vi "Encrypts.vi"(8 "error in (no error)":errorcluster caption="entrée d'erreur (pas d'erreur)", 11 "Cryptographic Hash_SHA256 en entrée":refnum<class "Cryptographic Hash_SHA256.lvclass">) -> (0 "error out":errorcluster caption="sortie d'erreur", 3 "Cryptographic Hash_SHA256 en sortie":refnum<class "Cryptographic Hash_SHA256.lvclass">)   [LabVIEW 2020, in "Library Cryptographic Hash.lvlib" / "Cryptographic Hash_SHA256.lvclass"]
uses:
  Cryptographic Hash_SHA256.lvclass
  C:/Users/ngarcin/OneDrive - Altyor/Standard TB/Class/Cryptographic Hash/Cryptographic Hash (Default)/Cryptographic Hash (Default).lvclass
  Cryptographic Hash_SHA256.lvclass/Cryptographic Hash_SHA256.ctl
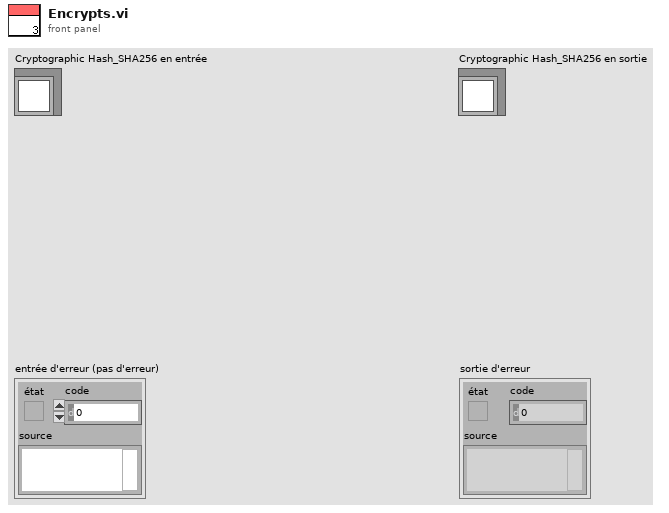
[diagram p1: front panel]
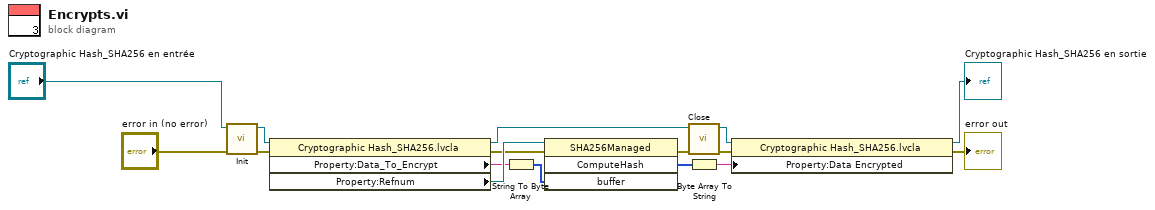
[diagram p0: block diagram]
diagram:
  n1 = call-dynamic "Init.vi"("error in (no error)"="error in (no error)", "Cryptographic Hash_SHA256 en entrée"="Cryptographic Hash_SHA256 en entrée") -> ("error out"=w12:errorcluster, "Cryptographic Hash_SHA256 en sortie"=w13:refnum<class "Cryptographic Hash_SHA256.lvclass">)  [unwired: 8 in]
  n2 = property class="Cryptographic Hash_SHA256.lvcla"(reference=w13, error in=w12) -> (reference out=w10:refnum<class "Cryptographic Hash_SHA256.lvclass">, error out=w2:errorcluster, "Property:Data_To_Encrypt"=w3:string, "Property:Refnum"=w4:refnum<k24>)
  n3 = String To Byte Array(string=w3) -> (unsigned byte array=w16:u8[])
  n4 = invoke class="SHA256Managed" method="ComputeHash"(reference=w4, error in=w2, "buffer"=w16) -> (error out=w1:errorcluster, "ComputeHash"=w15:u8[])  [unwired: 1 in, 2 out]
  n5 = call-dynamic "Close.vi"("error in (no error)"=w1, "Cryptographic Hash_SHA256 en entrée"=w10) -> ("error out"=w6:errorcluster, "Cryptographic Hash_SHA256 en sortie"=w9:refnum<class "Cryptographic Hash_SHA256.lvclass">)  [unwired: 8 in]
  n6 = Byte Array To String(unsigned byte array=w15) -> (string=w7:string)
  n7 = property class="Cryptographic Hash_SHA256.lvcla"(reference=w9, error in=w6, "Property:Data Encrypted"=w7) -> (reference out=→"Cryptographic Hash_SHA256 en sortie":refnum<class "Cryptographic Hash_SHA256.lvclass">, error out=→"error out":errorcluster)
